vi "Skip scheduled cell.vi"(8 "error in (no error)":errorcluster, 11 "Run Block in":refnum<class "Run Block.lvclass">) -> (0 "error out":errorcluster, 2 "Skipped Run":refnum<class "Run Instance.lvclass">, 3 "Run Block out":refnum<class "Run Block.lvclass">)   [LabVIEW 2020, in "CIRCUS_uServices.lvlib" / "Run Utilities.lvlib" / "Run Block.lvclass"]
uses:
  Run Block.lvclass
  Run Instance/Run Instance.lvclass
  Schedule/Schedule.lvclass
  Cell/Schedule Cell.lvclass
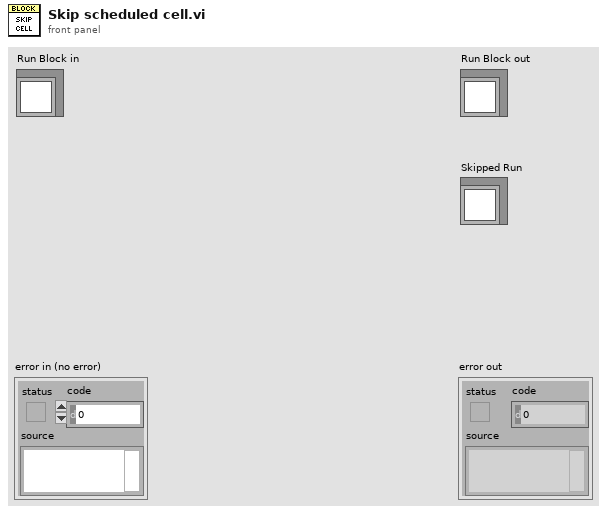
[diagram p1: front panel]
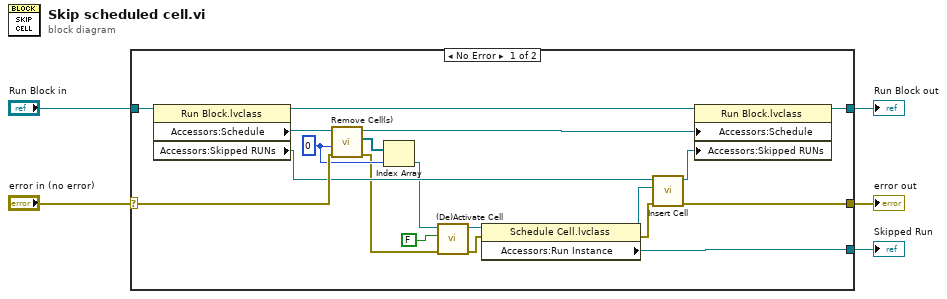
[diagram p0: block diagram]
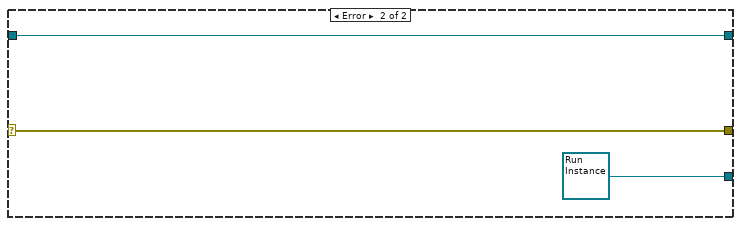
[diagram p2: hidden frame]
diagram:
  n1 = case shown="No Error" "error in (no error)" {
    selector: "error in (no error)" -> [w19 w27]
    tunnel: [w15 w27] -> w4
    tunnel: [w22 w26] -> w2
    tunnel: "Run Block in" -> [w24 w26]
    tunnel: [w13 refnum<class "Run Instance.lvclass"> refnum ("Run Instance")] -> w1
    frame No Error {
      w18 = 0 ("index")
      n2 = property class="Run Block.lvclass"(reference=w24) -> (reference out=w23:refnum<class "Run Block.lvclass">, "Accessors:Schedule"=w20:refnum<class "Schedule.lvclass">, "Accessors:Skipped RUNs"=w16:refnum<class "Schedule.lvclass">)  [unwired: 1 in, 1 out]
      n3 = call-dynamic "Remove Cell(s).vi"("error in (no error)"=w19, "index"=w18, "Schedule in"=w20) -> ("error out"=w10:errorcluster, "Deleted Cell(s)"=w17:refnum<class "Schedule Cell.lvclass">[], "Schedule out"=w21:refnum<class "Schedule.lvclass">)  [unwired: 6 in]
      n4 = Index Array(array=w17, index=w18) -> (element=w9:refnum<class "Schedule Cell.lvclass">)
      n5 = call-dynamic "(De)Activate Cell.vi"("error in (no error)"=w10, "Active"=FALSE, "Schedule Cell in"=w9) -> ("error out"=w7:errorcluster, "Schedule Cell out"=w8:refnum<class "Schedule Cell.lvclass">)  [unwired: 7 in]
      n6 = property class="Schedule Cell.lvclass"(reference=w8, error in=w7) -> (reference out=w12:refnum<class "Schedule Cell.lvclass">, error out=w11:errorcluster, "Accessors:Run Instance"=w13:refnum<class "Run Instance.lvclass">)
      n7 = call-dynamic "Insert Cell.vi"("error in (no error)"=w11, "Schedule Cell"=w12, "Schedule in"=w16) -> ("error out"=w15:errorcluster, "Schedule out"=w14:refnum<class "Schedule.lvclass">)  [unwired: 7 in]
      n8 = property class="Run Block.lvclass"(reference=w23, "Accessors:Schedule"=w21, "Accessors:Skipped RUNs"=w14) -> (reference out=w22:refnum<class "Run Block.lvclass">)  [unwired: 1 in, 1 out]
    }
    frame Error {
    }
  }
  "error out" <- w4
  "Run Block out" <- w2
  "Skipped Run" <- w1
